vi "Add Tree Nodes.vi"(6 "App Ref":refnum<vi>, 7 "Root path":string, 10 "Tree Map in":T1, 11 "Library In":refnum<class "Library.lvclass">) -> (2 "Tree Map out":T1, 3 "Library Out":refnum<class "Library.lvclass">)   [LabVIEW 2019, in "Panther Dashboard.lvlib"]
uses:
  Panther Dashboard.lvlib
  <vilib>/Delacor/Delacor QMH/Libraries/Scripting API/DQMH_Scripting API.lvlib
  <vilib>/Delacor/Delacor QMH/Libraries/_Scripting Support/Event Type (New)--enum.ctl
  <vilib>/Delacor/Delacor QMH/Libraries/_Scripting Support/dqmh_lib_DQMH Scripting Support.lvlib
  Class/Library/Library.lvclass
  <vilib>/National Instruments/Tree Map/Tree Map Data.ctl
  <vilib>/National Instruments/Tree Map/Tree Map.lvlib
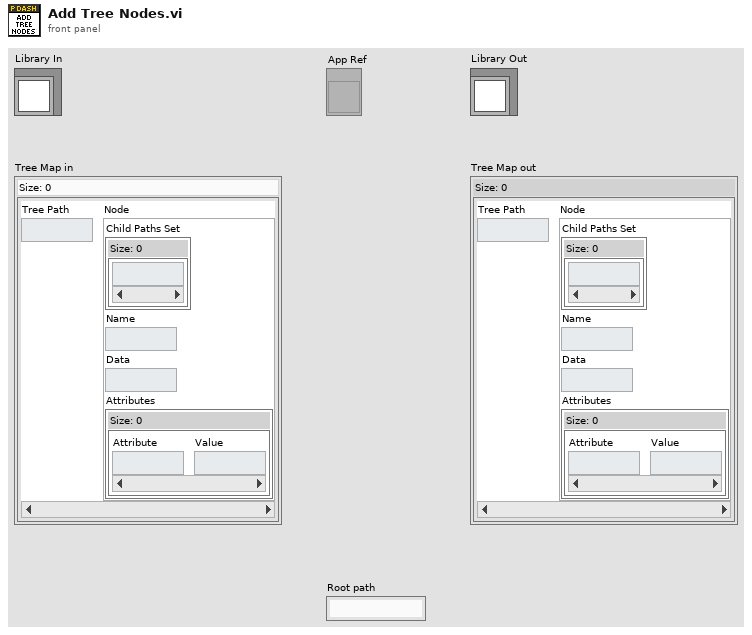
[diagram p1: front panel]
types:
  T1 = typedef "Tree Map.lvlib/Tree Map Data.ctl" = map{string, cluster{"Child Paths Set":set{string}, "Name":string, "Data":string, "Attributes":map{string, string}}}
  T2 = enum16{"Public API", "Constant VI", "Error VI"}[]
  T3 = typedef "dqmh_lib_DQMH Scripting Support.lvlib/Event Type (New)--enum.ctl" = enum16{"Request", "Broadcast", "Request and Wait for Reply", "Round Trip"}
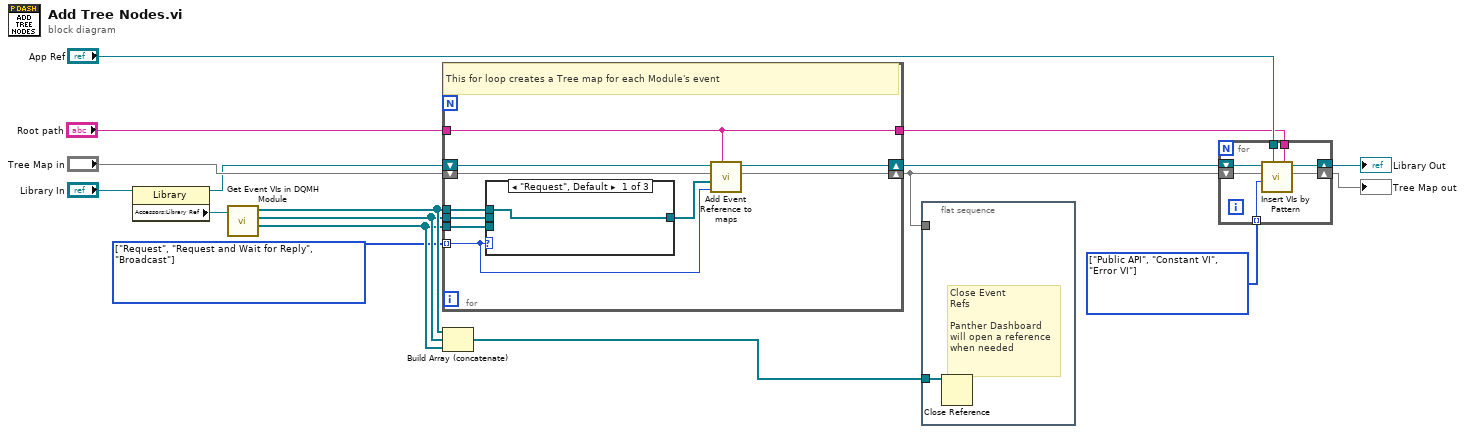
[diagram p0: block diagram]
diagram:
  w5 = T2 [enum."Public API", enum."Constant VI", enum."Error VI"] items=["Public API", "Constant VI", "Error VI"] ("Category")
  w10 = T3[] [enum."Request", enum."Request and Wait for Reply", enum."Broadcast"] items=["Request", "Broadcast", "Request and Wait for Reply", "Round Trip"] ("Event Type")
  n1 = property class="Library"(reference="Library In") -> (reference out=w7:refnum<class "Library.lvclass">, "Accessors:Library Ref"=w8:refnum<vi>)  [unwired: 1 in, 1 out]
  n2 = call <vilib>:"Get Event VIs in DQMH Module.vi"("DQMH Module"=w8) -> ("Broadcast Event VIs"=w13:refnum<vi>[], "Request and Wait for Reply Event VIs"=w14:refnum<vi>[], "Request Event VIs"=w15:refnum<vi>[])  [unwired: 7 in, 1 out]
  n3 = for {
    tunnel: w10 -> [w20] mode=indexing
    shift-right: [w25] -> w2
    shift-left: "Tree Map in" -> [w24]
    tunnel: w15 -> [w27]
    tunnel: w14 -> [w23]
    tunnel: w13 -> [w26]
    tunnel: "Root path" -> [w21]
    tunnel: [w21] -> w1
    shift-right: [w18] -> w3
    shift-left: w7 -> [w19]
    # "This for loop creates a Tree map for each Module's event"
    n4 = case shown="\"Request\", Default" w20 {
      tunnel: w27 -> [w28 _ _]
      tunnel: w26 -> [_ _ w30]
      tunnel: w23 -> [_ w29 _]
      tunnel: [w28 w29 w30] -> w22
      frame "Request", Default {
      }
      frame "Request and Wait for Reply" {
      }
      frame "Broadcast" {
      }
    }
    n5 = call "Add Event Reference to maps.vi"("Root Path"=w21, "Event Type"=w20, "Event VIs"=w22, "Tree Map in"=w24, "Library In"=w19) -> ("Tree Map out"=w25:T1, "Library Out"=w18:refnum<class "Library.lvclass">)  [unwired: 5 in]
  }
  n6 = Build Array (concatenate)(w15, w14, w13) -> (w12:refnum<vi>[])
  n7 = flat-sequence {
    tunnel: w2 -> [_]
    tunnel: w12 -> [w31]
    frame #0 {
      # "Close Event\nRefs\n\nPanther Dashboard\nwill open a reference\nwhen needed"
      n8 = Close Reference(reference=w31) -> ()  [unwired: 1 in, 1 out]
    }
  }
  n9 = for {
    tunnel: "App Ref" -> [w38]
    tunnel: w5 -> [w36] mode=indexing
    shift-right: [w37] -> w6
    shift-left: w3 -> [w34]
    shift-right: [w35] -> w4
    shift-left: w2 -> [w33]
    tunnel: w1 -> [w32]
    n10 = call "Insert VIs by Pattern.vi"("Root path"=w32, "Application in"=w38, "Category"=w36, "Tree Map in"=w33, "Library In"=w34) -> ("Tree Map Out"=w35:T1, "Library Out"=w37:refnum<class "Library.lvclass">)  [unwired: 5 in]
  }
  "Tree Map out" <- w4
  "Library Out" <- w6
